vi "CSM MDI Example.vi"() -> ()   [LabVIEW 2020]
uses:
  <userlib>/_NEVSTOP/Communicable State Machine(CSM)/_Support/GlobalEvent/GEvt-Convert Filter Rules - v1.0.vi
  MDI ViewManager/CSM MDI.vi
  <userlib>/_NEVSTOP/Communicable State Machine(CSM)/addons/INI-Static-Variable-Support/_Support/instances/_CSM - Read File Logger Configuration - v1.0.vi
  <userlib>/_NEVSTOP/Communicable State Machine(CSM)/addons/INI-Static-Variable-Support/_Support/instances/_CSM - Read Log Filter Rules - v1.0.vi
  <userlib>/_NEVSTOP/Communicable State Machine(CSM)/_Support/GlobalEvent/LogFilter/SettingVIs/Set Global CSM Filter.vi
  <userlib>/_NEVSTOP/Communicable State Machine(CSM)/_Support/GlobalEvent/LogFilter/SettingVIs/Set Global LogType Filter.vi
  <userlib>/_NEVSTOP/Communicable State Machine(CSM)/_Support/GlobalEvent/LogFilter/SettingVIs/Set Global State Filter.vi
  <userlib>/_NEVSTOP/Communicable State Machine(CSM)/_Support/GlobalEvent/LogFilter/SettingVIs/Set CSM LogType Filter.vi
  <userlib>/_NEVSTOP/Communicable State Machine(CSM)/_Support/GlobalEvent/LogFilter/SettingVIs/Set CSM State Filter.vi
  <userlib>/_NEVSTOP/Communicable State Machine(CSM)/_Support/GlobalEvent/LogFilter/SettingVIs/Set Global StateType Filter.vi
  <userlib>/_NEVSTOP/Communicable State Machine(CSM)/_Support/GlobalEvent/LogFilter/SettingVIs/Set CSM StateType Filter.vi
  <userlib>/_NEVSTOP/Communicable State Machine(CSM)/_Support/GlobalEvent/LogFilter/LogFilter.lvclass
  <userlib>/_NEVSTOP/Communicable State Machine(CSM)/Communicable State Machine.lvlib
  MDI ViewManager/MDI ViewManager.lvlib
  <userlib>/_NEVSTOP/Communicable State Machine(CSM)/addons/Watchdog/CSM Watchdog.lvlib
  <userlib>/_NEVSTOP/Communicable State Machine(CSM)/addons/INI-Static-Variable-Support/INI-Static-Variable-Support.lvlib
  <userlib>/_NEVSTOP/Communicable State Machine(CSM)/addons/Logger/CSM File Logger.lvlib
panel:
  out "Information":string="Load \"csm\"..."
  out "CSMVersion":string="Powered By CSM, Copyright ?2025 NEVSTOP-LAB"
  out "CSMScript(version)":string="CSM MDI Example"
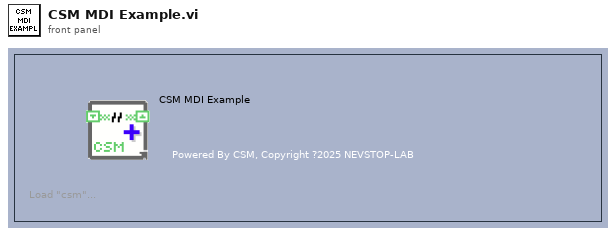
[diagram p1: front panel]
types:
  T1 = enum32{"Invalid", "Standard", "Closed", "Hidden", "Minimized", "Maximized"}
  T2 = cluster{"Enable":bool, "Limit":cluster{"FileSize":i64, "FileNum":i32}, "Timestamp.Format":string, "AutoExit":bool}
  T3 = typedef "Communicable State Machine.lvlib/_CSM_GlobalLog Filter Rules - v1.0.ctl" = cluster{"Global":cluster{"CSM":string[], "LogType":T4[], "State":string[], "StateType":T5[]}, "CSM":cluster{"LogType":cluster{"CSM":string, "LogType":T4}[], "State":cluster{"CSM":string, "State":string}[], "StateType":cluster{"CSM":string, "LogType":T5}[]}}
  T4 = typedef "Communicable State Machine.lvlib/_CSM_GlobalLog_MSG_TYPE.ctl" = enum16{"User Log", "State Change", "Status", "Interrupt", "Register", "Unregister", "Error Log", "Module Created", "Module Destroyed", "Async Message", "No-Rep Async Message", "Sync Message"}
  T5 = typedef "Communicable State Machine.lvlib/_CSM_GlobalLog_STATE_TYPE.ctl" = enum16{"State - Internal State", "State - External Message", "State - Response", "State - Complete"}
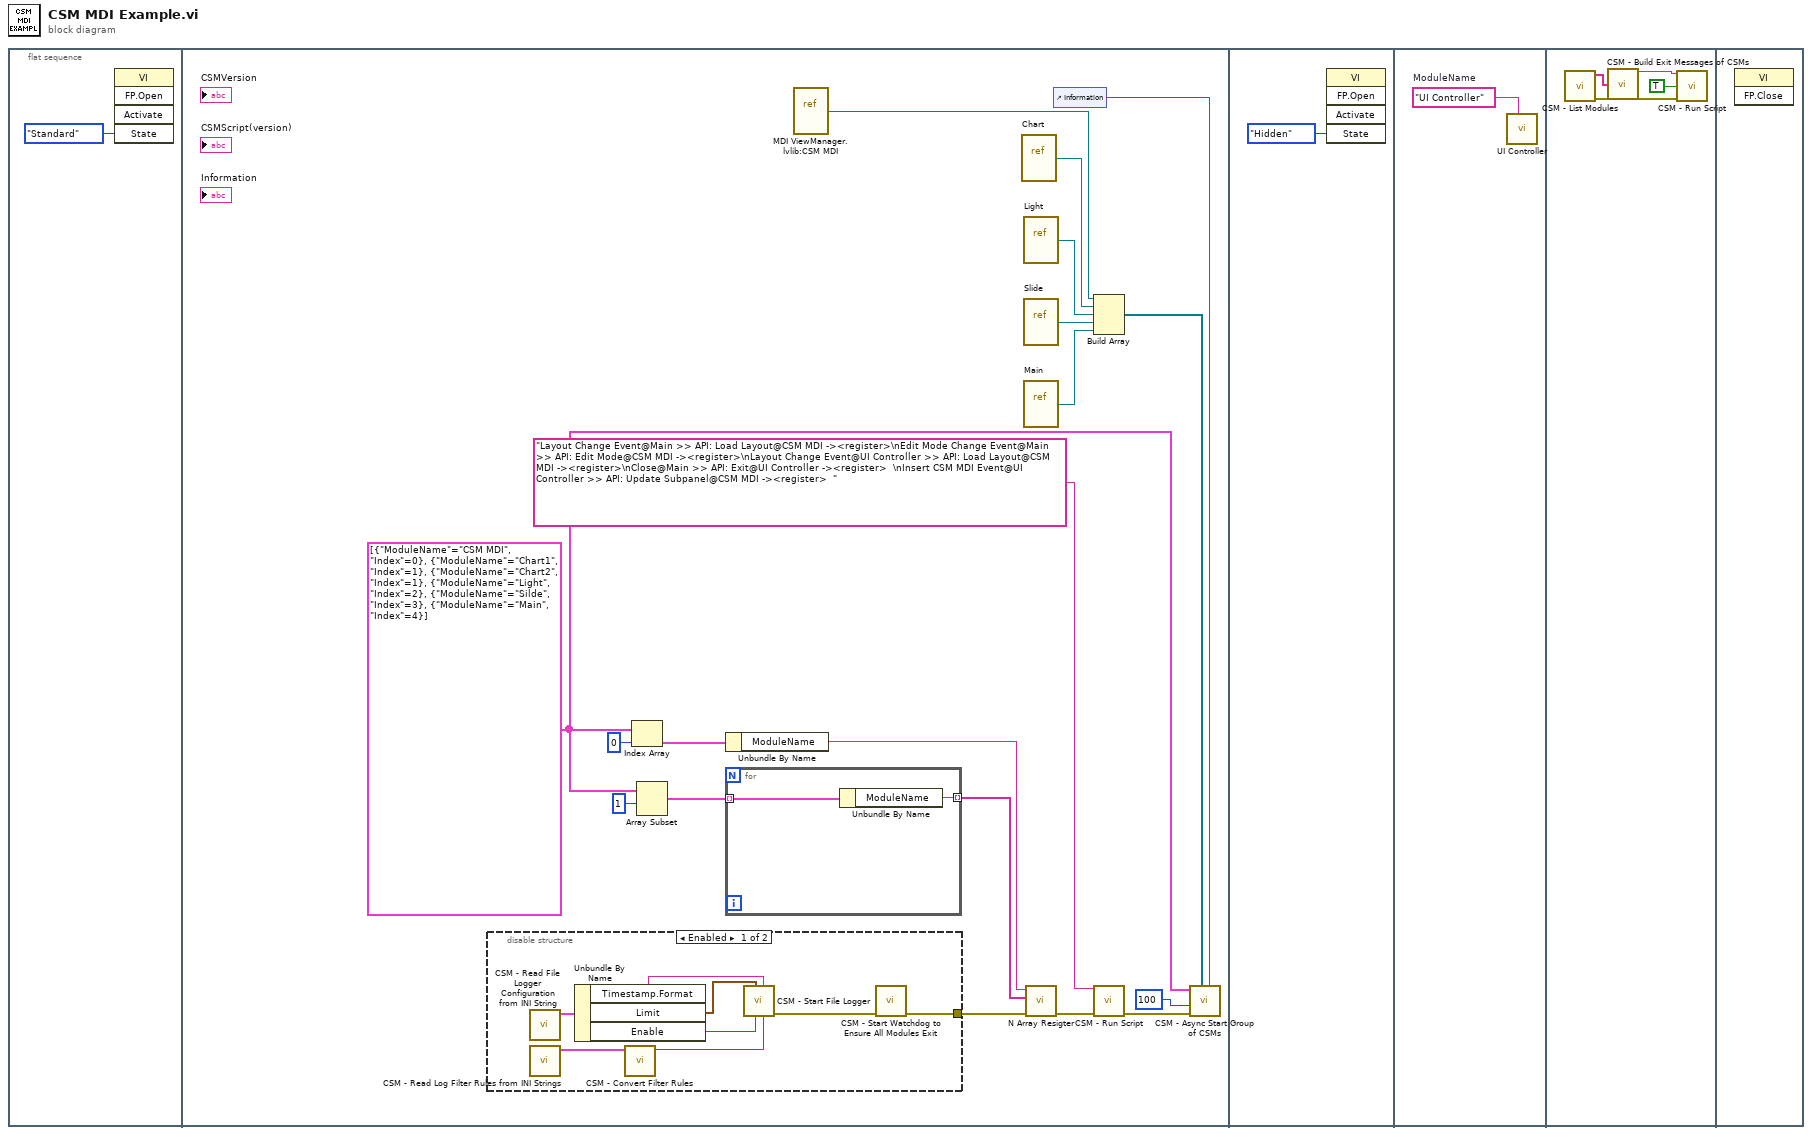
[diagram p0: block diagram]
diagram:
  n1 = flat-sequence {
    frame #0 {
      n2 = invoke class="VI" method="FP.Open"("State"=T1."Standard") -> ()  [unwired: 4 in, 5 out]
    }
    frame #1 {
      w14 = cluster{"ModuleName":string, "Index":i32}[] [{"ModuleName"="CSM MDI", "Index"=0}, {"ModuleName"="Chart1", "Index"=1}, {"ModuleName"="Chart2", "Index"=1}, {"ModuleName"="Light", "Index"=2}, {"ModuleName"="Silde", "Index"=3}, {"ModuleName"="Main", "Index"=4}]
      n3 = disable-structure shown="Enabled" {
        disable-tunnel: [w28 _] -> w12
        frame Enabled {
          n4 = call-poly <userlib>:"CSM - Read File Logger Configuration from INI String.vi"() -> ("FileLogger Configuration-v1"=w23:T2)  [unwired: 8 in, 1 out]
          n5 = call-poly <userlib>:"CSM - Read Log Filter Rules from INI Strings.vi"() -> ("Rules-v1"=w22:T3)  [unwired: 8 in, 1 out]
          n6 = Unbundle By Name(w23) -> ("Timestamp.Format"=w26:string, "Limit"=w25:cluster{"FileSize":i64, "FileNum":i32}, "Enable"=w24:bool)
          n7 = call-poly <userlib>:"CSM - Convert Filter Rules.vi"("Rules-v1"=w22) -> ("GlobalLogFilter"=w21:refnum<class "LogFilter.lvclass">)  [unwired: 10 in]
          n8 = call <userlib>:"CSM - Start File Logger.vi"("Filter Rules"=w21, "Timestamp Format"=w26, "Enable? (T)"=w24, "Log Limit"=w25) -> ("error out"=w27:errorcluster)  [unwired: 5 in, 2 out]
          n9 = call <userlib>:"CSM - Start Watchdog to Ensure All Modules Exit.vi"("error in (no error)"=w27) -> ("error out"=w28:errorcluster)  [unwired: 10 in]
        }
        frame Disabled {
        }
      }
      n10 = Index Array(array=w14, index=0) -> (element=w11:cluster{"ModuleName":string, "Index":i32})
      n11 = Array Subset(array=w14, index=1) -> (w10:cluster{"ModuleName":string, "Index":i32}[])  [unwired: 1 in]
      n12 = Unbundle By Name(w11) -> ("ModuleName"=w13:string)
      n13 = for {
        tunnel: w10 -> [w30] mode=indexing
        tunnel: [w29] -> w9 mode=indexing
        n14 = Unbundle By Name(w30) -> ("ModuleName"=w29:string)
      }
      n15 = vi-ref "MDI ViewManager.lvlib:CSM MDI.vi"() -> (w15:refnum<vi>)
      n16 = vi-ref "Chart.vi"() -> (w19:refnum<vi>)
      n17 = vi-ref "Light.vi"() -> (w18:refnum<vi>)
      n18 = vi-ref "Slide.vi"() -> (w17:refnum<vi>)
      n19 = vi-ref "Main.vi"() -> (w7:refnum<vi>)
      n20 = call "N Array Resigter.vi"("error in (no error)"=w12, "Event Source"=w9, "Taget"=w13) -> ("error out"=w5:errorcluster)  [unwired: 8 in]
      n21 = control-ref of="Information"() -> (w2:refnum<vi>)
      n22 = Build Array(w15, w19, w18, w17, w7) -> (w16:refnum<vi>[])
      n23 = call <userlib>:"CSM - Run Script.vi"("CSM Scripts"="Layout Change Event@Main >> API: Load Layout@CSM MDI -><register>\nEdit Mode Change Event@Main >> API: Edit Mode@CSM MDI -><register>\nLayout Change Event@UI Controller >> API: Load Layout@CSM MDI -><register>\nClose@Main >> API: Exit@UI Controller -><register>  \nInsert CSM MDI Event@UI Controller >> API: Update Subpanel@CSM MDI -><register>  ", "error in (no error)"=w5) -> ("error out"=w4:errorcluster)  [unwired: 11 in, 2 out]
      n24 = call "CSM - Async Start Group of CSMs.vi"("Information"=w2, "Prototypes"=w16, "error in (no error)"=w4, "interval(50ms)"=u32 100, "Module List"=w14) -> ()  [unwired: 4 in, 1 out]
    }
    frame #2 {
      n25 = invoke class="VI" method="FP.Open"("State"=T1."Hidden") -> ()  [unwired: 4 in, 5 out]
    }
    frame #3 {
      w32 = "UI Controller"  # ModuleName
      n26 = call "UI Controller.vi"("Name (\"\" to Use UUID)"=w32) -> ()  [unwired: 11 in]
    }
    frame #4 {
      n27 = call <userlib>:"CSM - List Modules.vi"() -> ("error out"=w35:errorcluster, "Module Names"=w33:string[])  [unwired: 10 in]
      n28 = call <userlib>:"CSM - Build Exit Messages of CSMs.vi"("CSMs"=w33) -> ("States"=w36:string)  [unwired: 14 in]
      n29 = call <userlib>:"CSM - Run Script.vi"("CSM Scripts"=w36, "Continue If Error? (F)"=TRUE, "error in (no error)"=w35) -> ()  [unwired: 10 in, 3 out]
    }
    frame #5 {
      n30 = invoke class="VI" method="FP.Close"() -> ()  [unwired: 3 in, 3 out]
    }
  }
